vi "Get Primary Destination Path.vi"(8 "error in (no error)":errorcluster, 11 "PPL in":refnum<class "NI_AB_API_PPL.lvclass">) -> (0 "error out":errorcluster, 2 "Primary destination path":path, 3 "PPL out":refnum<class "NI_AB_API_PPL.lvclass">)   [LabVIEW 2020, in "NI_AB_API_PPL.lvclass"]
uses:
  <vilib>/AppBuilder/AB_API/PPL/NI_AB_API_PPL.lvclass
  <vilib>/AppBuilder/AB_API/Targetfile/NI_AB_API_Targetfile.lvclass
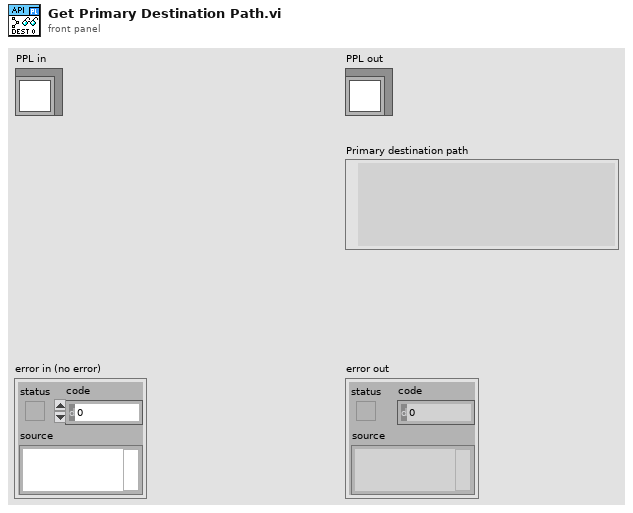
[diagram p1: front panel]
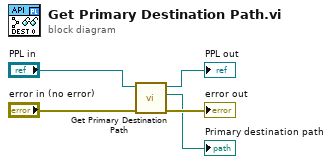
[diagram p0: block diagram]
diagram:
  n1 = call-parent "Get Primary Destination Path.vi"("error in (no error)"="error in (no error)", "NI_AB_API_Build in"="PPL in") -> ("error out"=→"error out":errorcluster, "Primary destination path"=→"Primary destination path":path, "NI_AB_API_Build out"=→"PPL out":refnum<class "NI_AB_API_PPL.lvclass">)  [unwired: 7 in]
